vi "down arrow.vi"() -> (3 "v":u8)   [LabVIEW 2021, in "AOC.lvlib"]
uses:
  AOC.lvlib
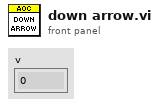
[diagram p1: front panel]
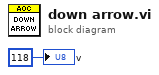
[diagram p0: block diagram]
diagram:
  "v" <- u8 118 ("element")
